vi "USBData_convert.vi"(7 "MeasurementIndex":i64, 8 "error in (no error)":errorcluster, 9 "LastDataAcquired":dbl[](array[numeric]), 10 "TimeMeasuremeent":timestamp, 11 "USBData in":refnum<class "USBData.lvclass">) -> (0 "error out":errorcluster, 1 "LeakDet_FULL":dbl format="%#_13g", 3 "USBData out":refnum<class "USBData.lvclass">, 5 "Status":T1(ring)=enum."Waiting")   [LabVIEW 2017, in "USBData.lvclass"]
uses:
  USBData.lvclass
  USBData.lvclass/USBData.ctl
  <vilib>/express/express arith-compare/Formula/XNode/ExpressFormulaBlockNode.xnode
panel:
  in  "Baratron_offset (defulat:0)":dbl format="%#_13g"
  out "LeakDet_Mantissa":dbl format="%#_13g"
  out "LeakDet_EXP":dbl format="%#_13g"
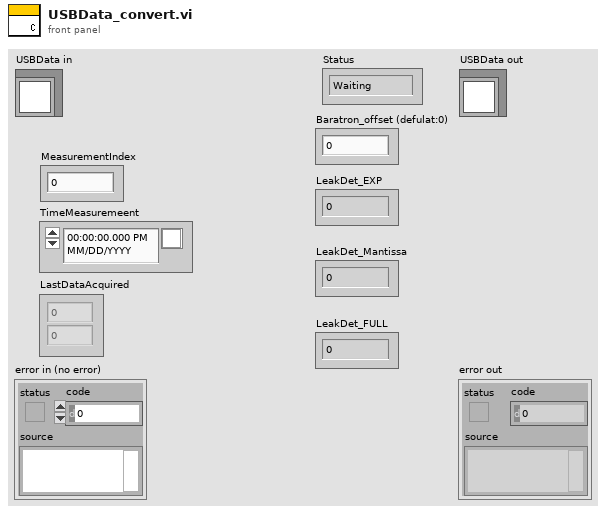
[diagram p1: front panel]
types:
  T1 = enum16{"Intialized", "Waiting", "Measuring", "Terminated"}
  T2 = cluster{"Type":enum16{"Raw", "SimpleProp", "CC-10_COMBINED", "CC-10_LOG", "LeakDet_EXP", "LeakDet_Mantissa", "Baratron"}, "ConversionParameters":dbl[]}[]
  T3 = enum16{"Raw", "SimpleProp", "CC-10_COMBINED", "CC-10_LOG", "LeakDet_EXP", "LeakDet_Mantissa", "Baratron"}
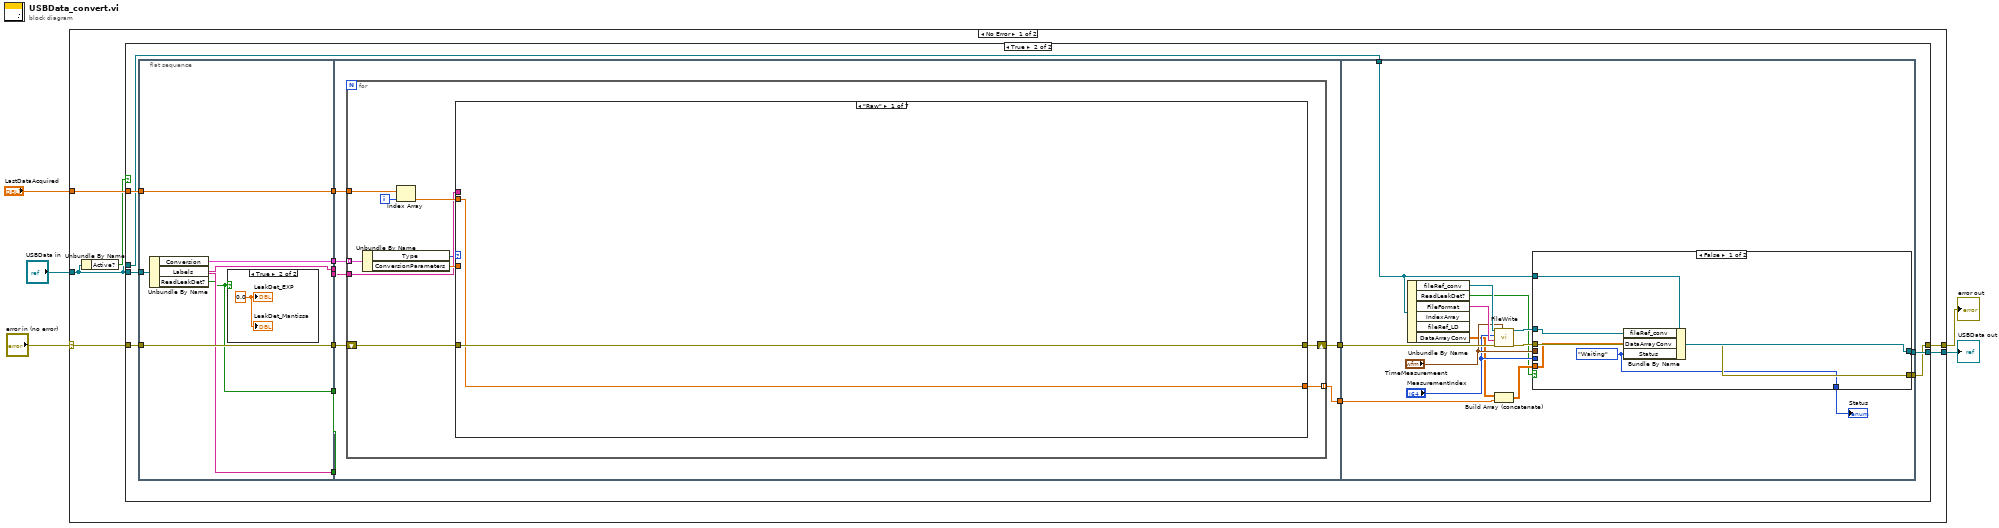
[diagram p0: block diagram]
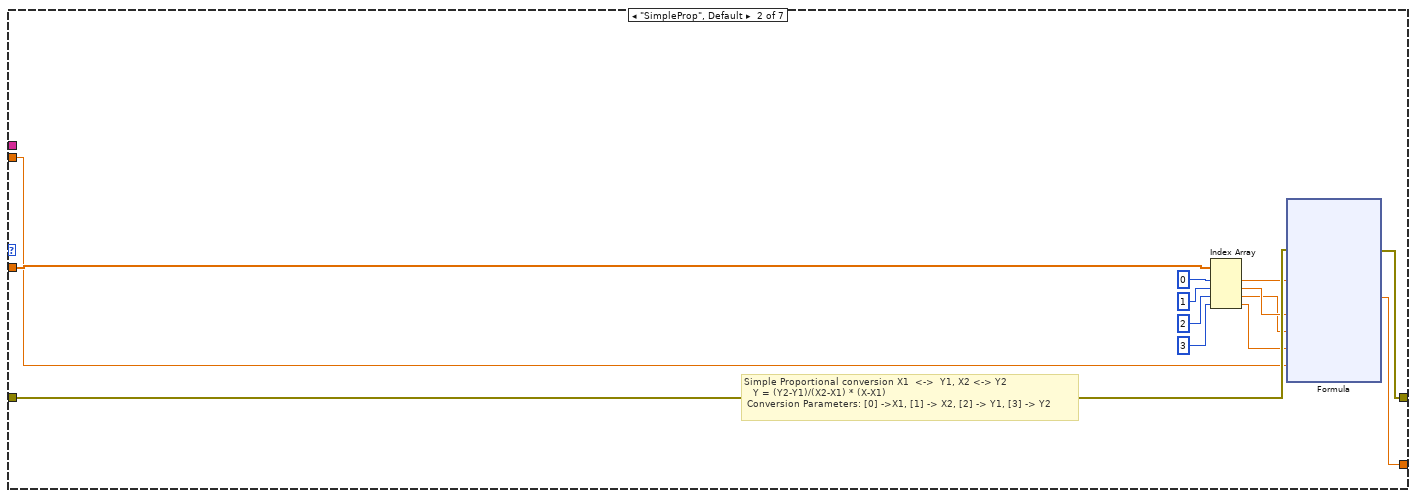
[diagram p4: hidden frame]
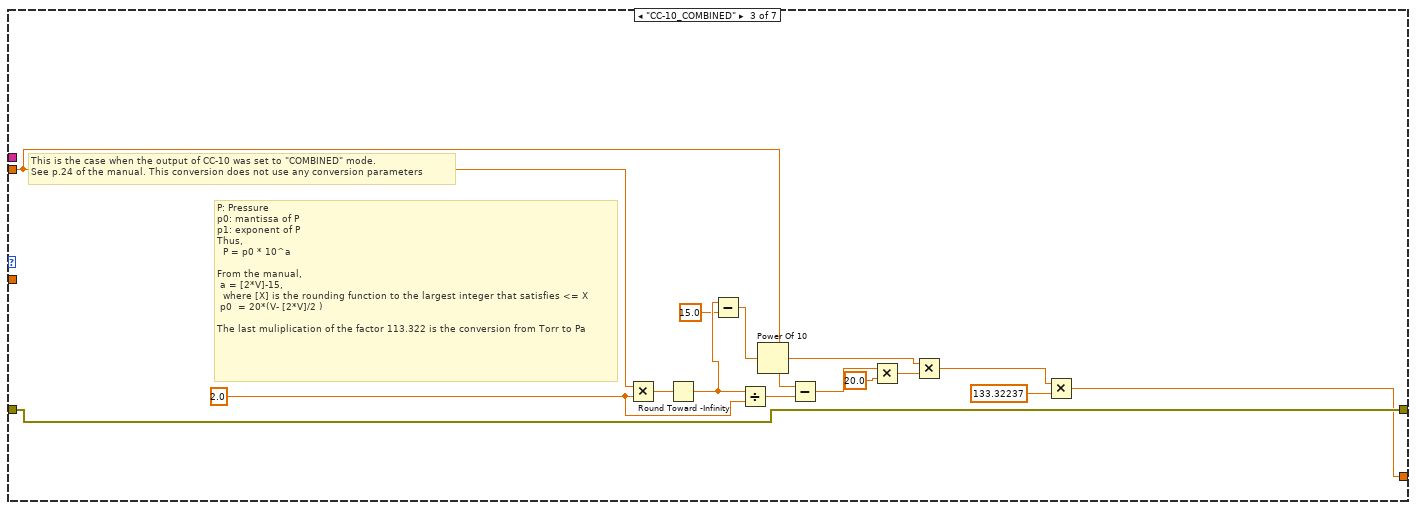
[diagram p5: hidden frame]
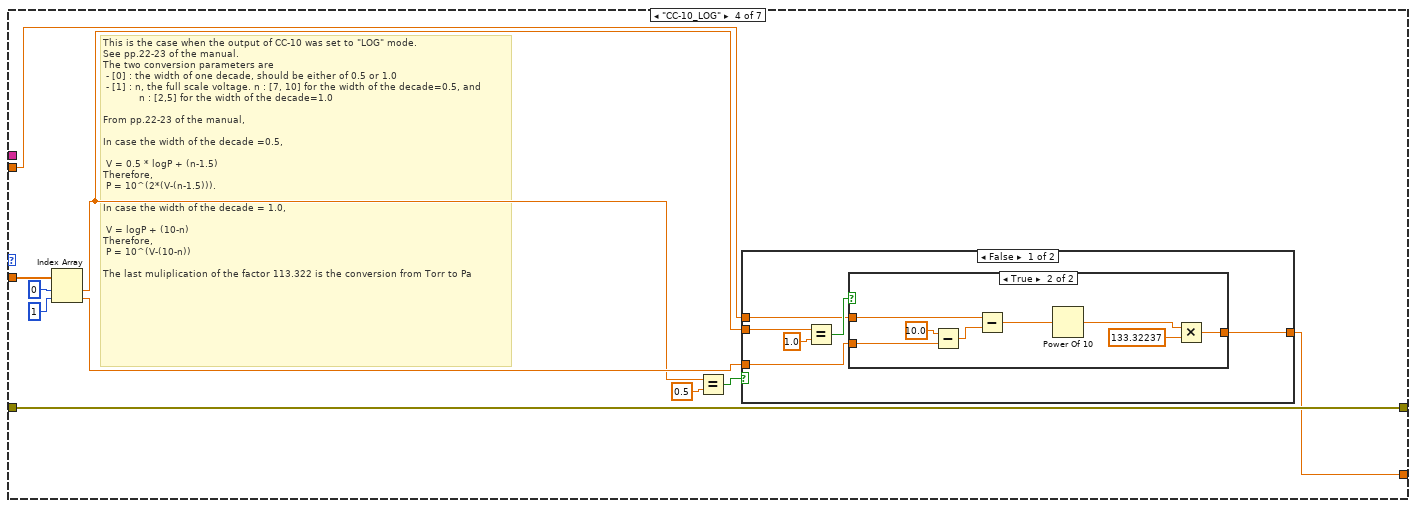
[diagram p6: hidden frame]
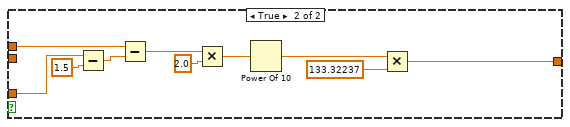
[diagram p8: hidden frame]
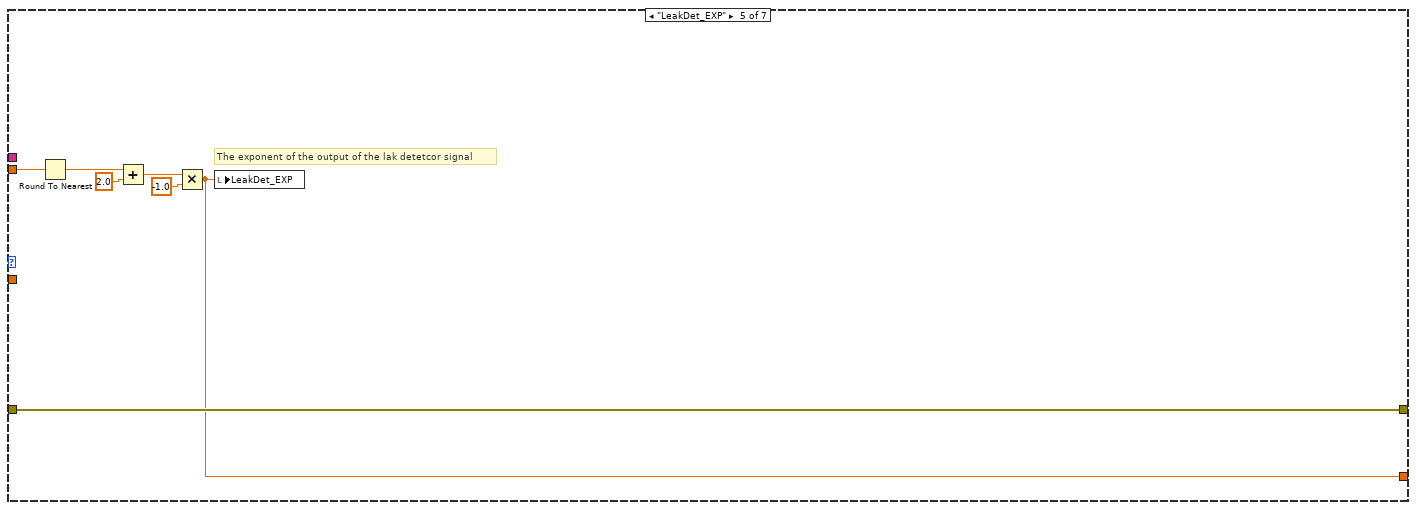
[diagram p9: hidden frame]
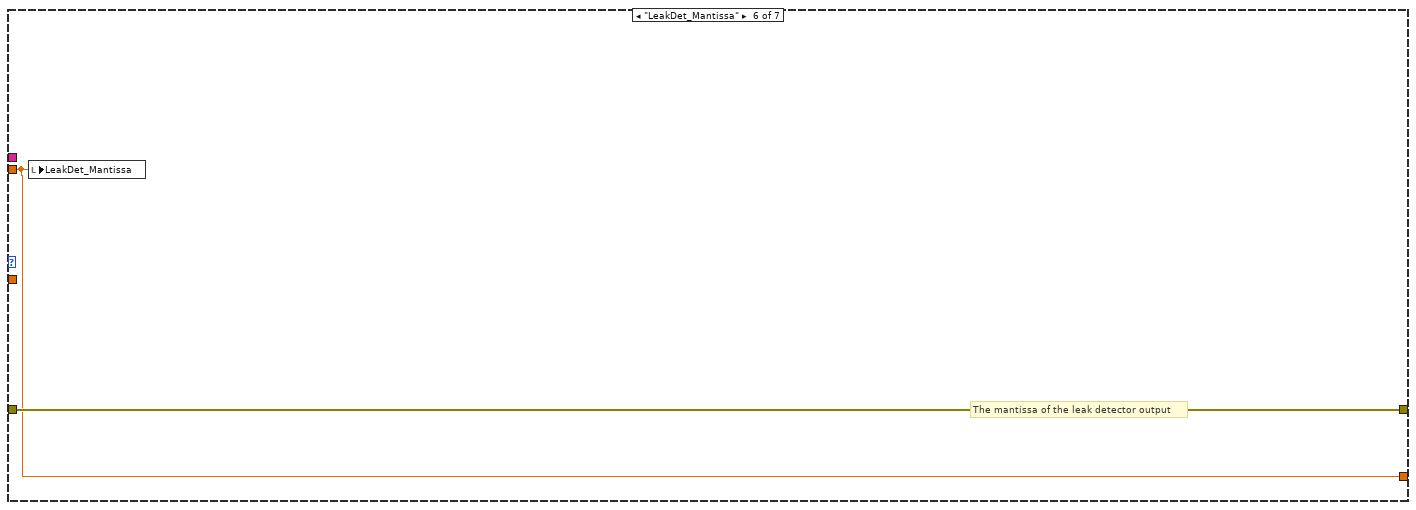
[diagram p10: hidden frame]
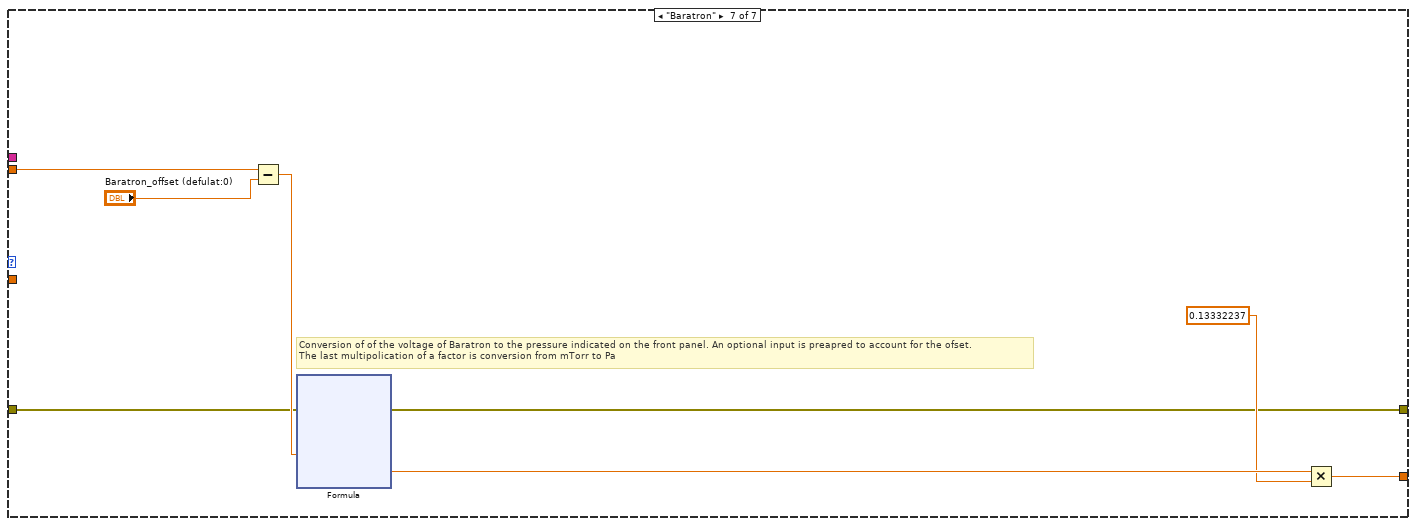
[diagram p11: hidden frame]
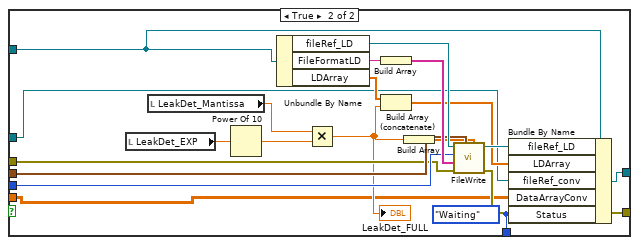
[diagram p12: hidden frame]
diagram:
  n1 = case shown="No Error" "error in (no error)" {
    selector: "error in (no error)" -> [w11 w199]
    tunnel: [w8 w199] -> w4
    tunnel: [w7 w198] -> w2
    tunnel: "USBData in" -> [w6 w198]
    tunnel: "LastDataAcquired" -> [w10 _]
    frame No Error {
      n2 = Unbundle By Name(w6) -> ("Active?"=w9:bool)
      n3 = case shown="True" w9 {
        tunnel: w6 -> [w12 w27]
        tunnel: w11 -> [w13 w26]
        tunnel: w10 -> [_ w25]
        tunnel: [w13 w15] -> w8
        tunnel: [w12 w16] -> w7
        tunnel: w6 -> [_ w17]
        frame False {
        }
        frame True {
          n4 = flat-sequence {
            tunnel: w25 -> [w31]
            tunnel: w26 -> [w32]
            tunnel: w27 -> [w33]
            tunnel: [w32] -> w24
            tunnel: [w31] -> w23
            tunnel: [w30] -> w22
            tunnel: [w29] -> w21
            tunnel: [w29] -> w20
            tunnel: [w28] -> w19
            tunnel: w24 -> [w40]
            tunnel: w23 -> [w39]
            tunnel: w22 -> [w38]
            tunnel: w21 -> [_]
            tunnel: w20 -> [w37]
            tunnel: w19 -> [_]
            tunnel: [w36] -> w18
            tunnel: [w35] -> w14
            tunnel: w18 -> [w170]
            tunnel: w17 -> [w162]
            tunnel: [w161] -> w16
            tunnel: [w159] -> w15
            tunnel: w14 -> [w157]
            frame #0 {
              n5 = Unbundle By Name(w33) -> ("Conversion"=w30:T2, "Labels"=w29:string[], "ReadLeakDet?"=w28:bool)
              n6 = case shown="True" w28 {
                frame False {
                }
                frame True {
                  w34 = 0.0 ("LeakDet_Mantissa")
                  "LeakDet_Mantissa" <- w34
                  "LeakDet_EXP" <- w34
                }
              }
            }
            frame #1 {
              n7 = for {
                tunnel: w39 -> [w49]
                tunnel: w38 -> [w44] mode=indexing
                tunnel: w37 -> [w45]
                shift-right: [w42] -> w36
                shift-left: w40 -> [w50]
                tunnel: [w41] -> w35 mode=indexing
                i -> [w48]
                n8 = Unbundle By Name(w44) -> ("Type"=w43:T3, "ConversionParameters"=w47:dbl[])
                n9 = Index Array(array=w49, index=w48) -> (element=w46:dbl)
                n10 = case shown="\"Raw\"" w43 {
                  tunnel: w47 -> [_ w60 _ w100 _ _ _]
                  tunnel: w50 -> [w52 w61 w86 w101 w133 w140 w143]
                  tunnel: w46 -> [w51 w55 w95 w102 w134 w139 w148]
                  tunnel: w45 -> [_ _ _ _ _ _ _]
                  tunnel: [w52 w54 w86 w101 w133 w140 w142] -> w42
                  tunnel: [w51 w53 w82 w97 w132 w139 w141] -> w41
                  frame "Raw" {
                  }
                  frame "SimpleProp", Default {
                    # "Simple Proportional conversion X1  <->  Y1, X2 <-> Y2\n   Y = (Y2-Y1)/(X2-X1) * (X-X1)\n Conversion Parameters: [0] ->X1, [1] -> X2, [2] -> Y1, [3] -> Y2"
                    n11 = Index Array(array=w60, index #1=0 ("index"), index #2=1 ("index"), index #3=2 ("index"), index #4=3 ("index")) -> (element #1=w59:dbl, element #2=w58:dbl, element #3=w57:dbl, element #4=w56:dbl)
                    n12 = xnode "Formula"("X1"=w59, "X2"=w58, "Y1"=w57, "Y2"=w56, "XX"=w55, "error in (no error)"=w61) -> ("Result"=w53:dbl, "error out"=w54:errorcluster)
                  }
                  frame "CC-10_COMBINED" {
                    w94 = 2.0 ("Numeric")
                    # "P: Pressure \np0: mantissa of P\np1: exponent of P\nThus,\n  P = p0 * 10^a\n\nFrom the manual, \n a = [2*V]-15, \n  where [X] is the rounding function to the largest integer that satisfies <= X \n p0  = 20*(V- [2*V]/2 )\n\nThe last muliplication of the factor 113.322 is the conversion from Torr to Pa"
                    # "This is the case when the output of CC-10 was set to \"COMBINED\" mode. \nSee p.24 of the manual. This conversion does not use any conversion parameters"
                    n13 = Multiply(x=w95, y=w94) -> (x*y=w96:dbl)
                    n14 = Round Toward -Infinity(1:w96) -> (0:w85:dbl)
                    n15 = Subtract(x=w85, y=15.0) -> (x-y=w84:dbl)
                    n16 = Divide(x=w85, y=w94) -> (x/y=w93:dbl)
                    n17 = Power Of 10(x=w84) -> (10^x=w89:dbl)
                    n18 = Subtract(x=w95, y=w93) -> (x-y=w92:dbl)
                    n19 = Multiply(x=w92, y=20.0 ("Numeric")) -> (x*y=w90:dbl)
                    n20 = Multiply(x=w89, y=w90) -> (x*y=w88:dbl)
                    n21 = Multiply(x=w88, y=133.32237) -> (x*y=w82:dbl)
                  }
                  frame "CC-10_LOG" {
                    # "This is the case when the output of CC-10 was set to \"LOG\" mode. \nSee pp.22-23 of the manual. \nThe two conversion parameters are\n - [0] : the width of one decade, should be either of 0.5 or 1.0\n - [1] : n, the full scale voltage. n : [7, 10] for the width of the decade=0.5, and \n            n : [2,5] for the width of the decade=1.0\n\nFrom pp.22-23 of the manual,\n\nIn case the width of the decade =0.5,\n\n V = 0.5 * logP + (n-1.5)\nTherefore,\n P = 10^(2*(V-(n-1.5))).\n\nIn case the width of the decade = 1.0,\n\n V = logP + (10-n)\nTherefore,\n P = 10^(V-(10-n))\n\nThe last muliplication of the factor 113.322 is the conversion from Torr to Pa"
                    n22 = Index Array(array=w100, index #1=0 ("index"), index #2=1 ("index")) -> (element #1=w98:dbl, element #2=w99:dbl)
                    n23 = Equal?(x=w98, y=0.5) -> (x = y?=w103:bool)
                    n24 = case shown="False" w103 {
                      tunnel: w102 -> [w110 w129]
                      tunnel: [w109 w124] -> w97
                      tunnel: w99 -> [w108 w122]
                      tunnel: w98 -> [w107 _]
                      frame False {
                        n25 = Equal?(x=w107, y=1.0) -> (x = y?=w111:bool)
                        n26 = case shown="True" w111 {
                          tunnel: w110 -> [w113 w119]
                          tunnel: [w113 w115] -> w109
                          tunnel: w108 -> [_ w114]
                          frame False {
                          }
                          frame True {
                            n27 = Subtract(x=10.0 ("y"), y=w114) -> (x-y=w120:dbl)
                            n28 = Subtract(x=w119, y=w120) -> (x-y=w118:dbl)
                            n29 = Power Of 10(x=w118) -> (10^x=w116:dbl)
                            n30 = Multiply(x=w116, y=133.32237) -> (x*y=w115:dbl)
                          }
                        }
                      }
                      frame True {
                        n31 = Subtract(x=w122, y=1.5) -> (x-y=w128:dbl)
                        n32 = Subtract(x=w129, y=w128) -> (x-y=w127:dbl)
                        n33 = Multiply(x=w127, y=2.0) -> (x*y=w126:dbl)
                        n34 = Power Of 10(x=w126) -> (10^x=w123:dbl)
                        n35 = Multiply(x=w123, y=133.32237) -> (x*y=w124:dbl)
                      }
                    }
                  }
                  frame "LeakDet_EXP" {
                    # "The exponent of the output of the lak detetcor signal"
                    n36 = Round To Nearest(number=w134) -> (nearest integer value=w135:dbl)
                    n37 = Add(x=w135, y=2.0) -> (x+y=w137:dbl)
                    n38 = Multiply(x=w137, y=-1.0) -> (x*y=w132:dbl)
                    n39 = local write "LeakDet_EXP"(w132) -> ()
                  }
                  frame "LeakDet_Mantissa" {
                    # "The mantissa of the leak detector output"
                    n40 = local write "LeakDet_Mantissa"(w139) -> ()
                  }
                  frame "Baratron" {
                    # "Conversion of of the voltage of Baratron to the pressure indicated on the front panel. An optional input is preapred to account for the ofset.\nThe last multipolication of a factor is conversion from mTorr to Pa"
                    n41 = Subtract(x=w148, y="Baratron_offset (defulat:0)") -> (x-y=w146:dbl)
                    n42 = xnode "Formula"("X"=w146, "error in (no error)"=w143) -> ("Result"=w145:dbl, "error out"=w142:errorcluster)
                    n43 = Multiply(x=w145, y=0.13332237) -> (x*y=w141:dbl)
                  }
                }
              }
            }
            frame #2 {
              n44 = Unbundle By Name(w162) -> ("fileRef_conv"=w169:refnum<file>, "ReadLeakDet?"=w160:bool, "FileFormat"=w171:string[], "DataArrayConv"=w165:dbl[][])  [unwired: 2 out]
              n45 = call "FileWrite.vi"("Time Stamp"="TimeMeasuremeent", "Error In"=w170, "FileFormat"=w171, "Index"="MeasurementIndex", "refnum in"=w169) -> ("Error Out"=w166:errorcluster, "Byte Stream File Refnum"=w164:refnum<file>)  [unwired: 5 in]
              n46 = Build Array (concatenate)(w165, w157) -> (w163:dbl[][])
              n47 = case shown="False" w160 {
                tunnel: "TimeMeasuremeent" -> [_ w195]
                tunnel: "MeasurementIndex" -> [_ w190]
                tunnel: w166 -> [w174 w189]
                tunnel: w162 -> [w177 w183]
                tunnel: w164 -> [w176 w184]
                tunnel: w163 -> [w172 w178]
                tunnel: [w175 w182] -> w161
                tunnel: [w174 w181] -> w159
                tunnel: [w173 w180] -> w158
                frame False {
                  w173 = T1."Waiting" ("Status")
                  n48 = Bundle By Name(cluster=w177, "fileRef_conv"=w176, "DataArrayConv"=w172, "Status"=w173) -> (w175:refnum<class "USBData.lvclass">)
                }
                frame True {
                  w180 = T1."Waiting" ("Status")
                  n49 = local read "LeakDet_EXP"() -> (w193:dbl)
                  n50 = local read "LeakDet_Mantissa"() -> (w194:dbl)
                  n51 = Power Of 10(x=w193) -> (10^x=w192:dbl)
                  n52 = Unbundle By Name(w183) -> ("fileRef_LD"=w196:refnum<file>, "FileFormatLD"=w187:string, "LDArray"=w186:dbl[])
                  n53 = Multiply(x=w194, y=w192) -> (x*y=w179:dbl)
                  "LeakDet_FULL" <- w179
                  n54 = Build Array(w187) -> (w197:string[])
                  n55 = Build Array (concatenate)(w186, w179) -> (w185:dbl[])
                  n56 = Build Array(w179) -> (w191:dbl[])
                  n57 = call "FileWrite.vi"("DataArray"=w191, "Time Stamp"=w195, "Error In"=w189, "FileFormat"=w197, "Index"=w190, "refnum in"=w196) -> ("Error Out"=w181:errorcluster, "Byte Stream File Refnum"=w188:refnum<file>)  [unwired: 4 in]
                  n58 = Bundle By Name(cluster=w183, "fileRef_LD"=w188, "LDArray"=w185, "fileRef_conv"=w184, "DataArrayConv"=w178, "Status"=w180) -> (w182:refnum<class "USBData.lvclass">)
                }
              }
              "Status" <- w158
            }
          }
        }
      }
    }
    frame Error {
    }
  }
  "error out" <- w4
  "USBData out" <- w2
